vi "Picture to Map.vi"(11 "path to JPEG file":path=path "C:/Users/Carl/Desktop/Untitled.png") -> (2 "Map out":bool[][](array[boolean]))   [LabVIEW 2020]
uses:
  SubVIs/Read-Only Globals.vi
  SubVIs/Globals (private).vi
  Square/Square.lvclass
panel:
  out "24-bit pixmap 2":u32[][](array[numeric]) format="%.0x"
  out "24-bit pixmap":u32[][](array[numeric]) format="%.0x"
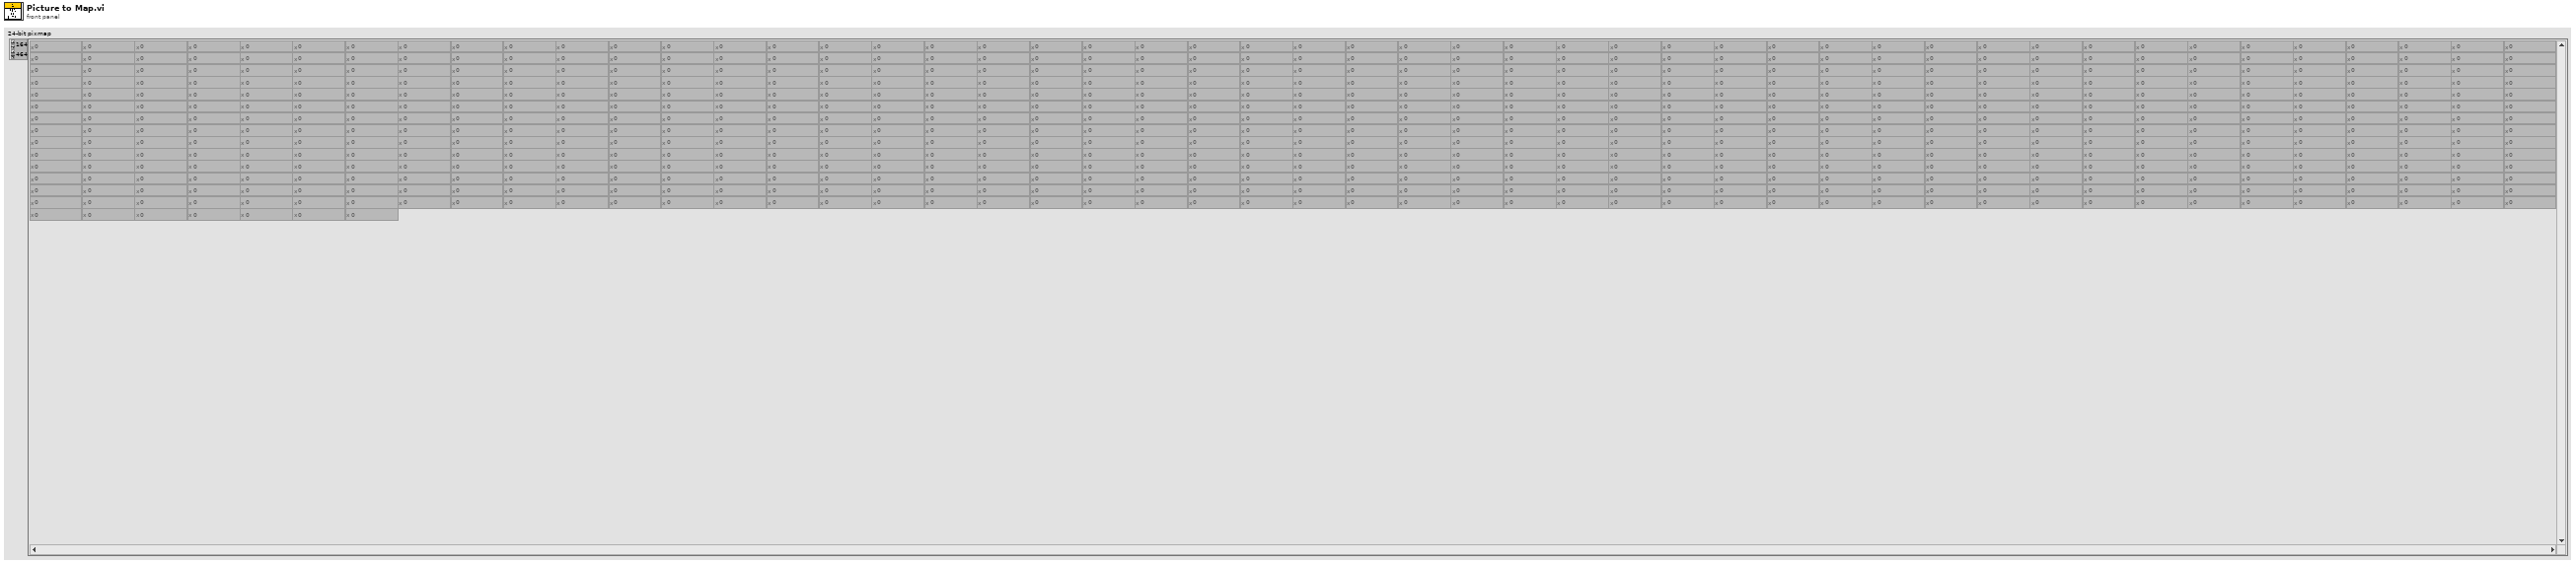
[diagram p1: front panel]
types:
  T1 = typedef "imagedata.ctl" = cluster{"image type":i32, "image depth":i32, "image":u8[], "mask":u8[], "colors":u32[], "Rectangle":cluster{"left":i16, "top":i16, "right":i16, "bottom":i16}}
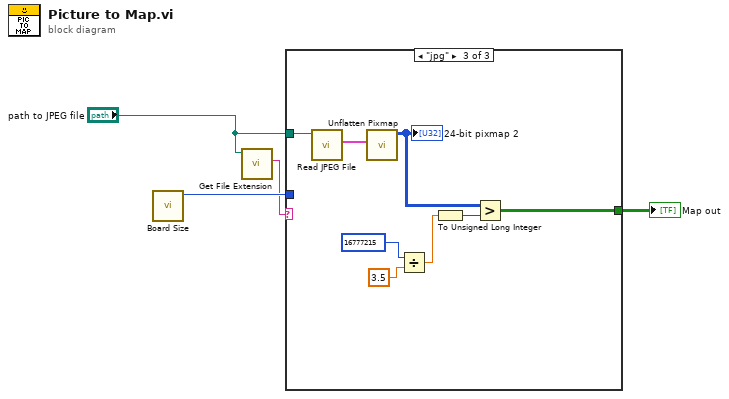
[diagram p0: block diagram]
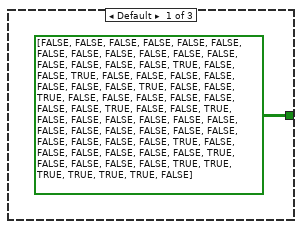
[diagram p2: hidden frame]
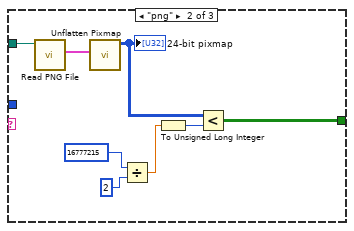
[diagram p3: hidden frame]
diagram:
  n1 = call "Board Size.vi"() -> ("Board Size"=w3:i32)  [unwired: 11 in]
  n2 = call <vilib>:"Get File Extension.vi"("file"="path to JPEG file") -> ("lowercase file extension"=w1:string)  [unwired: 6 in, 4 out]
  n3 = case shown="\"jpg\"" w1 {
    tunnel: "path to JPEG file" -> [_ w13 w21]
    tunnel: [bool[][] [[FALSE, FALSE, FALSE, FALSE, FALSE, FALSE, FALSE, FALSE, FALSE, FALSE, FALSE], [FALSE, FALSE, FALSE, FALSE, FALSE, TRUE, FALSE, FALSE, TRUE, FALSE, FALSE], [FALSE, FALSE, FALSE, FALSE, FALSE, TRUE, FALSE, FALSE, TRUE, FALSE, FALSE], [FALSE, FALSE, FALSE, FALSE, FALSE, TRUE, FALSE, FALSE, TRUE, FALSE, FALSE], [FALSE, FALSE, FALSE, FALSE, FALSE, FALSE, FALSE, FALSE, FALSE, FALSE, FALSE], [FALSE, FALSE, FALSE, TRUE, FALSE, FALSE, FALSE, FALSE, FALSE, FALSE, TRUE], [FALSE, FALSE, FALSE, FALSE, TRUE, TRUE, TRUE, TRUE, TRUE, TRUE, FALSE]] ("Map in") w10 w18] -> w4
    tunnel: w3 -> [_ _ _]
    frame Default {
    }
    frame "png" {
      n4 = call <vilib>:"Read PNG File.vi"("path to PNG file"=w13) -> ("image data"=w12:T1)  [unwired: 8 in, 2 out]
      n5 = call <vilib>:"Unflatten Pixmap.vi"("image data"=w12) -> ("24-bit pixmap"=w11:u32[][])  [unwired: 4 in, 6 out]
      "24-bit pixmap" <- w11
      n6 = Divide(x=u32 16777215, y=u32 2) -> (x/y=w7:dbl)
      n7 = To Unsigned Long Integer(number=w7) -> (unsigned 32bit integer=w6:u32)
      n8 = Less?(x=w11, y=w6) -> (x < y?=w10:bool[][])
    }
    frame "jpg" {
      n9 = call <vilib>:"Read JPEG File.vi"("path to JPEG file"=w21) -> ("image data"=w20:T1)  [unwired: 8 in, 2 out]
      n10 = call <vilib>:"Unflatten Pixmap.vi"("image data"=w20) -> ("24-bit pixmap"=w19:u32[][])  [unwired: 4 in, 6 out]
      "24-bit pixmap 2" <- w19
      n11 = Divide(x=u32 16777215, y=3.5) -> (x/y=w15:dbl)
      n12 = To Unsigned Long Integer(number=w15) -> (unsigned 32bit integer=w14:u32)
      n13 = Greater?(x=w19, y=w14) -> (0:w18:bool[][])
    }
  }
  "Map out" <- w4
